vi "Get Client Rectangle.vi"(8 "error in":errorcluster caption="error in (no error)" {"code" format="%d\n%x"}, 11 "window refnum (NaWR)":T1) -> (0 "error out":errorcluster {"code" format="%d\n%x"}, 2 "client rect":T2, 3 "window refnum out":T1)   [LabVIEW 2020, in "MacroAssert.lvlib" / "Win Util New.lvlib"]
doc: "This VI will find the coordinates of the upper left and lower right corners of the window identified by the 'window refnum' parameter. Coordinate values are in pixels, relative to the upper left corner of the screen. The 'window refnum' can be obtained by using 'Get Window RefNum.vi'."
uses:
  Win Util New.lvlib
  Window Refnum.ctl
  kernel32.dll
  user32.dll
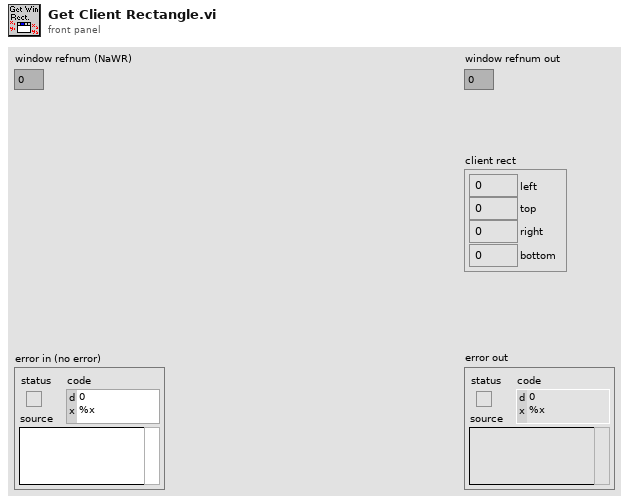
[diagram p1: front panel]
types:
  T1 = typedef "MacroAssert.lvlib/Win Util New.lvlib/Window Refnum.ctl" = u64
  T2 = cluster{"left":i16, "top":i16, "right":i16, "bottom":i16}
  T3 = cluster{"RECT[0]":i32, "RECT[1]":i32, "RECT[2]":i32, "RECT[3]":i32}
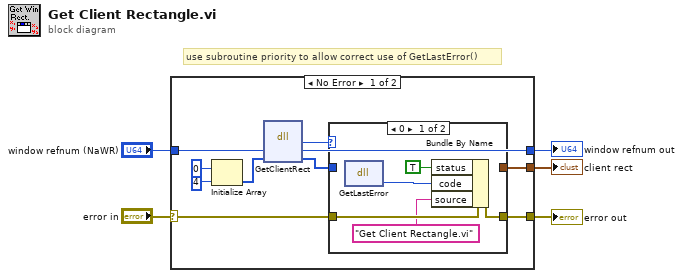
[diagram p0: block diagram]
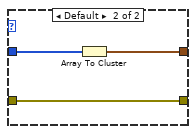
[diagram p2: hidden frame]
diagram:
  # "use subroutine priority to allow correct use of GetLastError()"
  n1 = case shown="No Error" "error in" {
    selector: "error in" -> [w7 w25]
    tunnel: [w9 w24] -> w3
    tunnel: [w6 w25] -> w5
    tunnel: "window refnum (NaWR)" -> [w10 w24]
    tunnel: [w11 _] -> w2
    frame No Error {
      n2 = Initialize Array(0, 4) -> (w13:i32[])
      n3 = dll-call lib="USER32.DLL" fn="GetClientRect"("hWnd"=w10, "RECT"=w13) -> ("Return Value"=w8:i32, "hWnd"=w9:u64, "RECT"=w12:i32[])  [unwired: 3 in, 2 out]
      n4 = case shown="0" w8 {
        tunnel: w12 -> [_ w23]
        tunnel: [_ w22] -> w11
        tunnel: w7 -> [w20 w21]
        tunnel: [w19 w21] -> w6
        frame 0 {
          n5 = dll-call lib="kernel32.dll" fn="GetLastError"() -> ("return type"=w17:i32)  [unwired: 3 in, 2 out]
          n6 = Bundle By Name(cluster=w20, "status"=TRUE ("show call chain? (False)"), "code"=w17, "source"="Get Client Rectangle.vi") -> (w19:errorcluster)
        }
        frame Default {
          n7 = Array To Cluster(array=w23) -> (cluster=w22:T3)
        }
      }
    }
    frame Error {
    }
  }
  "error out" <- w5
  "window refnum out" <- w3
  "client rect" <- w2
